vi "Timer_Stop.vi"(8 "Pass_Through_Time":dbl=-1.0 format="%33.4f", 11 "in Timer":T1 {"Accumulated TIme" format="%13.5p"; "StartTime" format="%13.5p"}) -> (3 "out Timer":T1 {"Accumulated TIme" format="%13.5p"; "StartTime" format="%13.5p"})   [LabVIEW 2019, in "Trajectory_Library.lvlib"]
doc: "Stop the timer. This computes the time as of now and clears the running flag, causing all subsequent time requests to be read from the accumulated time rather than looking at the system clock.\n\nInputs:\n - Timer -- The Timer data cluster\n\nOutputs:\n - Timer -- The modified Timer data cluster"
uses:
  Trajectory_Library.lvlib
  TypeDef/TIMER.ctl
  Timer_GetInternal.vi
  Util_GetTime.vi
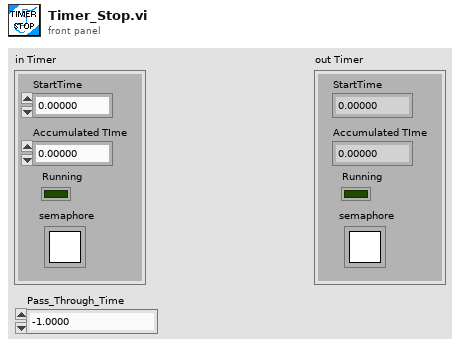
[diagram p1: front panel]
types:
  T1 = typedef "Trajectory_Library.lvlib/TIMER.ctl" = cluster{"StartTime":dbl, "Accumulated TIme":dbl, "Running":bool, "semaphore":T2}
  T2 = typedef "Semaphore RefNum" = refnum<k1>
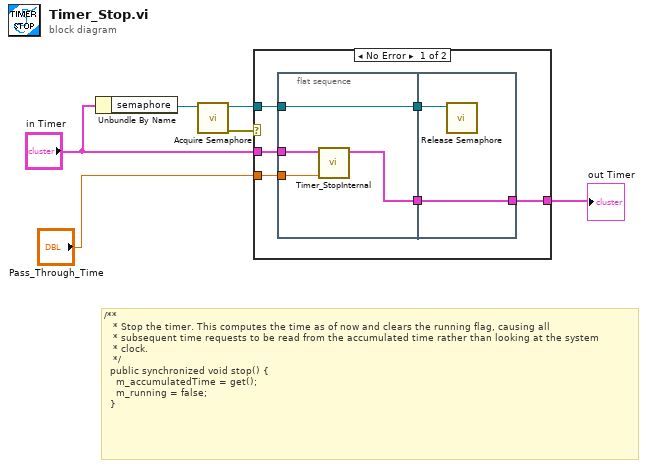
[diagram p0: block diagram]
diagram:
  # "/**\n   * Stop the timer. This computes the time as of now and clears the running flag, causing all\n   * subsequent time requests to be read from the accumulated time rather than looking at the system\n   * clock.\n   */\n  public synchronized void stop() {\n    m_accumulatedTime = get();\n    m_running = false;\n  }"
  n1 = Unbundle By Name("in Timer") -> ("semaphore"=w5:T2)
  n2 = call <vilib>:"Acquire Semaphore.vi"("semaphore"=w5) -> ("error out"=w3:errorcluster, "semaphore out"=w2:T2)  [unwired: 4 in, 1 out]
  n3 = case shown="No Error" w3 {
    tunnel: [w12 w19] -> w6
    tunnel: "in Timer" -> [w11 w19]
    tunnel: w2 -> [w8 _]
    tunnel: "Pass_Through_Time" -> [w7 _]
    frame No Error {
      n4 = flat-sequence {
        tunnel: w11 -> [w15]
        tunnel: [w16] -> w10
        tunnel: [w14] -> w9
        tunnel: w8 -> [w14]
        tunnel: w7 -> [w13]
        tunnel: [w18] -> w12
        tunnel: w10 -> [w18]
        tunnel: w9 -> [w17]
        frame #0 {
          n5 = call "Timer_StopInternal.vi"("Pass_Through_Time"=w13, "in Timer"=w15) -> ("out Timer"=w16:T1)  [unwired: 9 in]
        }
        frame #1 {
          n6 = call <vilib>:"Release Semaphore.vi"("semaphore"=w17) -> ()  [unwired: 5 in, 2 out]
        }
      }
    }
    frame Error {
    }
  }
  "out Timer" <- w6
